vi "LabVIEW Version To Year.vi"(0 "LabVIEW Version":string) -> (2 "LabVIEW Year":u32)   [LabVIEW 2019, in "VIPM.lvlib" / "VIPM Item.lvclass"]
uses:
  VIPM Item.lvclass
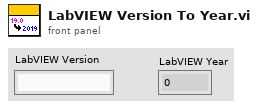
[diagram p1: front panel]
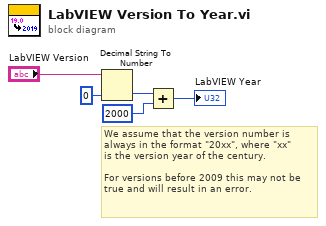
[diagram p0: block diagram]
diagram:
  # "We assume that the version number is\nalways in the format \"20xx\", where \"xx\"\nis the version year of the century.\n\nFor versions before 2009 this may not be\ntrue and will result in an error."
  n1 = Decimal String To Number(string="LabVIEW Version", default (0L)=u32 0 ("default (0 I32)")) -> (number=w4:u32)  [unwired: 1 in, 1 out]
  n2 = Add(x=w4, y=u32 2000) -> (x+y=→"LabVIEW Year":u32)
